vi "Handle.vi"(11 "Ex Event Actor in":refnum<class "Ex Event Actor.lvclass">) -> (2 "Destroy?":bool, 3 "Ex Event Actor out":refnum<class "Ex Event Actor.lvclass">)   [LabVIEW 2021, in "Ex Event Actor.lvlib" / "Ex Event Actor.lvclass"]
uses:
  Ex Event Actor.lvclass
  Ex Event Actor.lvclass/Ex Event Actor.ctl
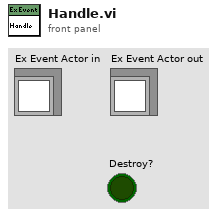
[diagram p1: front panel]
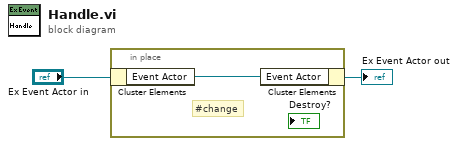
[diagram p0: block diagram]
diagram:
  n1 = in-place {
    # "#change"
    n2 = in-place-cluster #1("Ex Event Actor in") -> ("Event Actor"=w3:refnum<class "Event Actor.lvclass">)
    n3 = in-place-cluster #1("Event Actor"=w3) -> (→"Ex Event Actor out":refnum<class "Ex Event Actor.lvclass">)
  }
